vi "Export To Spreadsheet String.vi"(0 "XYGraph":refnum<vi>, 7 "Scale":dbl) -> (8 "spreadsheet string":string)   [LabVIEW 2020, in "Interactive Graph.xctl"]
uses:
  Interactive Graph.xctl
  Math VIs/LinSpace (x0-dx-npts).vi
  <vilib>/Analysis/baseanly.llb/Mean (DBL).vi
  Array Manipulation VIs/Irregular Array Subset (DBL).vi
  <vilib>/Analysis/NI_AALBase.lvlib
panel:
  out "error out":errorcluster
  in  "error in (no error)":errorcluster
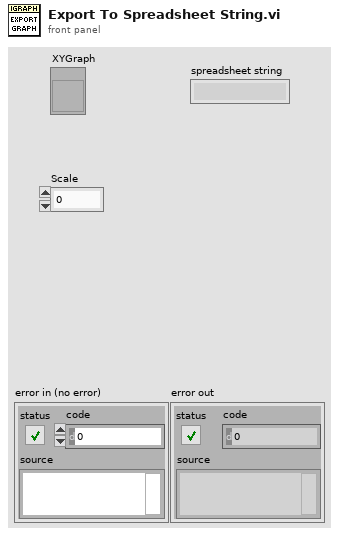
[diagram p1: front panel]
types:
  T1 = typedef "LVAnnotationListTypeDef.ctl" = cluster{"Name":string, "Color":u32, "Style":u8, "Point Style":u8, "Name Visible":bool, "Allow Drag":bool, "Annotation Mode":u32, "Plot":i32, "Index":i32, "Position":cluster{"X":dbl, "Y":dbl}, "X Scale":u32, "Y Scale":u32, "Show Arrow":bool, "Lock Name":bool, "Plot Area":i32, "Label Offset":cluster{"X":dbl, "Y":dbl}}[]
  T2 = cluster{"Array Subset":dbl[], dbl[], "Name":string}
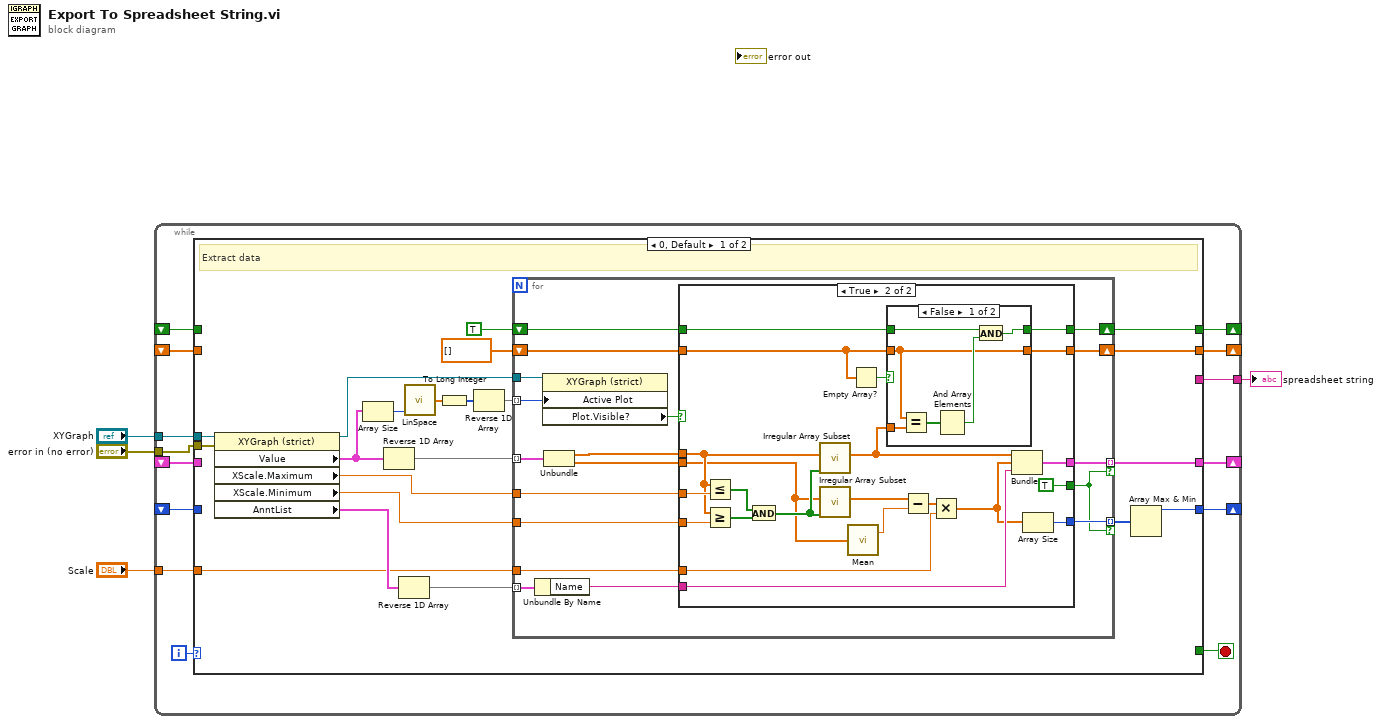
[diagram p0: block diagram]
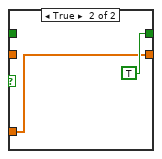
[diagram p3: hidden frame]
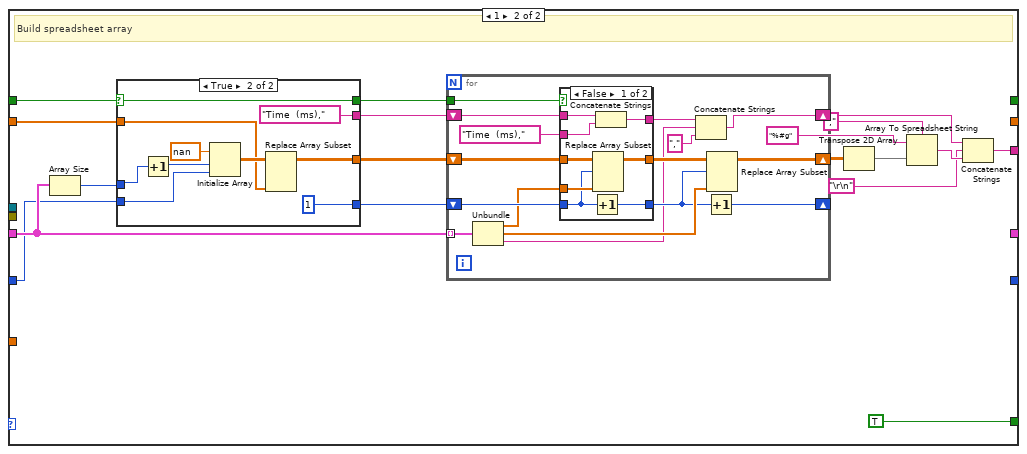
[diagram p4: hidden frame]
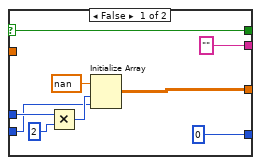
[diagram p6: hidden frame]
diagram:
  n1 = while {
    tunnel: "XYGraph" -> [w18]
    tunnel: "error in (no error)" -> [w17]
    shift-right: [w14] -> _
    shift-left: _ -> [w10]
    shift-right: [w13] -> _
    shift-left: _ -> [w9]
    shift-right: [w12] -> _
    shift-left: _ -> [w8]
    shift-right: [w11] -> _
    shift-left: _ -> [w7]
    tunnel: [w6] -> w2
    tunnel: "Scale" -> [w5]
    i -> [w16]
    stop <- w15 stop-if-true
    n2 = case shown="0, Default" w16 {
      tunnel: w18 -> [w37 _]
      tunnel: w17 -> [w36 _]
      tunnel: [_ TRUE] -> w15
      tunnel: [w31 _] -> w14
      tunnel: [w30 _] -> w13
      tunnel: [w29 _] -> w12
      tunnel: [w28 _] -> w11
      tunnel: w10 -> [_ w102]
      tunnel: w9 -> [_ w104]
      tunnel: w8 -> [_ w103]
      tunnel: w7 -> [_ w105]
      tunnel: [_ w93] -> w6
      tunnel: w5 -> [w19 _]
      frame 0, Default {
        # "Extract data"
        n3 = property class="XYGraph (strict)"(reference=w37, error in=w36) -> (reference out=w27:refnum<vi>, "Value"=w23:cluster{dbl[], dbl[]}[], "XScale.Maximum"=w38:dbl, "XScale.Minimum"=w39:dbl, "AnntList"=w35:T1)  [unwired: 1 out]
        n4 = Array Size(array=w23) -> (size(s)=w24:i32)
        n5 = Reverse 1D Array(array=w23) -> (reversed array=w26:cluster{dbl[], dbl[]}[])
        n6 = Reverse 1D Array(array=w35) -> (reversed array=w25:T1)
        n7 = call-poly "LinSpace.vi"("npts"=w24) -> ("Array"=w22:dbl[])  [unwired: 3 in, 1 out]
        n8 = To Long Integer(number=w22) -> (32bit integer=w20:i32[])
        n9 = Reverse 1D Array(array=w20) -> (reversed array=w21:i32[])
        n10 = for {
          tunnel: w26 -> [w45] mode=indexing
          tunnel: w38 -> [w57]
          tunnel: w39 -> [w56]
          tunnel: w25 -> [w55] mode=indexing
          shift-right: [w52] -> w29
          shift-left: dbl[] [] -> [w53]
          shift-right: [w51] -> w28
          shift-left: TRUE -> [w54]
          tunnel: [w50] -> w30 mode=indexing if=w44
          tunnel: [w49] -> w32 mode=indexing if=w44
          tunnel: w27 -> [w41]
          tunnel: w21 -> [w43] mode=indexing
          tunnel: w19 -> [w40]
          n11 = Unbundle By Name(w55) -> ("Name"=w46:string)
          n12 = property class="XYGraph (strict)"(reference=w41, "Active Plot"=w43) -> ("Plot.Visible?"=w42:bool)  [unwired: 1 in, 2 out]
          n13 = Unbundle(w45) -> (w48:dbl[], w47:dbl[])
          n14 = case shown="True" w42 {
            tunnel: w57 -> [_ w81]
            tunnel: w56 -> [_ w80]
            tunnel: w48 -> [_ w77]
            tunnel: w47 -> [_ w64]
            tunnel: w54 -> [w59 w75]
            tunnel: w53 -> [w58 w73]
            tunnel: [w59 w74] -> w51
            tunnel: [w58 w71] -> w52
            tunnel: [_ w69] -> w50
            tunnel: [_ TRUE] -> w44
            tunnel: w46 -> [_ w67]
            tunnel: [_ w66] -> w49
            tunnel: w40 -> [_ w60]
            frame False {
            }
            frame True {
              n15 = Less Or Equal?(x=w77, y=w81) -> (x <= y?=w79:bool[])
              n16 = Greater Or Equal?(x=w77, y=w80) -> (x >= y?=w78:bool[])
              n17 = And(x=w79, y=w78) -> (x .and. y?=w76:bool[])
              n18 = call-poly "Irregular Array Subset.vi"("Mask"=w76, "Array"=w77) -> ("Array Subset"=w70:dbl[])  [unwired: 8 in, 1 out]
              n19 = call-poly "Irregular Array Subset.vi"("Mask"=w76, "Array"=w64) -> ("Array Subset"=w65:dbl[])  [unwired: 8 in, 1 out]
              n20 = call-poly <vilib>:"Mean.vi"("X"=w64) -> ("mean"=w62:dbl)  [unwired: 1 out]
              n21 = Empty Array?(array=w73) -> (empty?=w72:bool)
              n22 = case shown="False" w72 {
                tunnel: w70 -> [w87 w88]
                tunnel: w75 -> [w86 _]
                tunnel: [w85 TRUE] -> w74
                tunnel: w73 -> [w82 _]
                tunnel: [w82 w88] -> w71
                frame False {
                  n23 = Equal?(x=w82, y=w87) -> (x = y?=w84:bool[])
                  n24 = And Array Elements(Boolean array=w84) -> (logical AND=w83:bool)
                  n25 = And(x=w86, y=w83) -> (x .and. y?=w85:bool)
                }
                frame True {
                }
              }
              n26 = Subtract(x=w65, y=w62) -> (x-y=w63:dbl[])
              n27 = Multiply(x=w63, y=w60) -> (x*y=w61:dbl[])
              n28 = Bundle("Array Subset"=w70, w61, "Name"=w67) -> (w69:T2)  [unwired: 1 in]
              n29 = Array Size(array=w61) -> (size(s)=w66:i32)
            }
          }
        }
        n30 = Array Max & Min(array=w32) -> (max value=w31:i32)  [unwired: 3 out]
      }
      frame 1 {
        # "Build spreadsheet array"
        n31 = Array Size(array=w104) -> (size(s)=w106:i32)
        n32 = case shown="True" w105 {
          selector: w105 -> [w138 w147]
          tunnel: w106 -> [w143 w145]
          tunnel: w103 -> [_ w149]
          tunnel: w102 -> [w135 w144]
          tunnel: [w140 w150] -> w101
          tunnel: [0 1] -> w100
          tunnel: [w138 w147] -> w99
          tunnel: ["" "Time  (ms),"] -> w98
          frame False {
            n33 = Multiply(x=w143, y=2) -> (x*y=w136:i32)
            n34 = Initialize Array(nan ("element"), w136, w135) -> (w140:dbl[][])
          }
          frame True {
            n35 = Increment(x=w145) -> (x+1=w152:i32)
            n36 = Initialize Array(nan ("element"), w152, w144) -> (w151:dbl[][])
            n37 = Replace Array Subset(array=w151, new element=w149) -> (w150:dbl[][])  [unwired: 2 in]
          }
        }
        n38 = for {
          tunnel: w104 -> [w123] mode=indexing
          shift-right: [w115] -> _
          shift-left: w100 -> [w122]
          tunnel: w99 -> [w121]
          shift-right: [w114] -> w97
          shift-left: w101 -> [w120]
          shift-right: [w110] -> w92
          shift-left: w98 -> [w113]
          n39 = Unbundle(w123) -> ("Array Subset"=w119:dbl[], w117:dbl[], "Name"=w109:string)
          n40 = case shown="False" w121 {
            tunnel: w122 -> [w129 w133]
            tunnel: w120 -> [w131 w134]
            tunnel: w119 -> [w130 _]
            tunnel: [w128 w134] -> w118
            tunnel: [w127 w133] -> w116
            tunnel: w113 -> [w126 w132]
            tunnel: "Time  (ms)," -> [w125 _]
            tunnel: [w124 w132] -> w111
            frame False {
              n41 = Increment(x=w129) -> (x+1=w127:i32)
              n42 = Replace Array Subset(array=w131, new element=w130, index (row)=w129) -> (w128:dbl[][])  [unwired: 1 in]
              n43 = Concatenate Strings(w126, w125) -> (w124:string)
            }
            frame True {
            }
          }
          n44 = Concatenate Strings(w111, w109, ",") -> (w110:string)
          n45 = Increment(x=w116) -> (x+1=w115:i32)
          n46 = Replace Array Subset(array=w118, new element=w117, index (row)=w116) -> (w114:dbl[][])  [unwired: 1 in]
        }
        n47 = Transpose 2D Array(2D array=w97) -> (transposed array=w96:dbl[][])
        n48 = Array To Spreadsheet String(delimiter (Tab)=",", array=w96, 3:"%#g" ("format string")) -> (spreadsheet string=w94:string)
        n49 = Concatenate Strings(w92, "\r\n", w94) -> (w93:string)
      }
    }
  }
  "spreadsheet string" <- w2
